vi "CoreDac.vi"(11 "Cluster":T1) -> ()   [LabVIEW 2024]
uses:
  #AquisitionLoopEnum.ctl
  <vilib>/DAQmx/create/channels.llb/DAQmx Create Channel (AI-Voltage-Basic).vi
  <vilib>/DAQmx/configure/timing.llb/DAQmx Timing (Sample Clock).vi
  <vilib>/DAQmx/read.llb/DAQmx Read (Analog 1D Wfm NChan NSamp).vi
  GUI/#GuiEnum.ctl
  GUI/#GuiQueueElement.ctl
  vision/#QueueEnum.ctl
  Correlation/#CorrelationQueueElement.ctl
  <vilib>/vision/Image Controls.llb/IMAQ Image.ctl
  Core/#CoreQueues.ctl
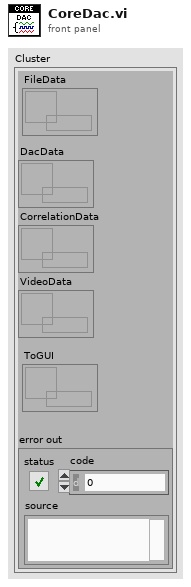
[diagram p1: front panel]
types:
  T1 = typedef "#CoreQueues.ctl" = cluster{"DacData":refnum<queue>, "CorrelationData":refnum<queue>, "VideoData":refnum<queue>, "error out":errorcluster, "ToGUI":refnum<queue>, "FileData":refnum<queue>}
  T2 = typedef "#AquisitionLoopEnum.ctl" = enum16{"Idle", "Init", "Aquisition", "End"}
  T3 = typedef "#QueueEnum.ctl" = enum16{"Ant", "Video"}
  T4 = typedef "#CorrelationQueueElement.ctl" = cluster{"Enum":T3, "t0":timestamp, dbl[]}
  T5 = typedef "#GuiEnum.ctl" = enum16{"AudioData", "VisionDistances", "DacDistances", "CorrelationDistances", "Video", "FPS"}
  T6 = typedef "#GuiQueueElement.ctl" = cluster{"Enum":T5, "Variant":variant}
  T7 = typedef "#AquisitionParameter.ctl" = cluster{"SampleRate":dbl, "BufferSize":i32, "Channels":tag}
  T8 = typedef "Sound Data Format.ctl" = cluster{"sample rate (S/s)":dbl, "number of channels":i32, "bits per sample":i32}
  T9 = cluster{"AquisitionParameters":T7, "SoundFormat":T8, "Signal type":enum16{"Sine Wave", "Triangle Wave", "Square Wave", "Sawtooth Wave"}, "Amplitude":dbl, "AudioBuffer":i32, "ChannelBounds":cluster{"InputMin":dbl, "InputMax":dbl, "OutputMin":dbl, "OutputMax":dbl}[], "MasterOffset":dbl}
  T10 = cluster{"InputMin":dbl, "InputMax":dbl, "OutputMin":dbl, "OutputMax":dbl}[]
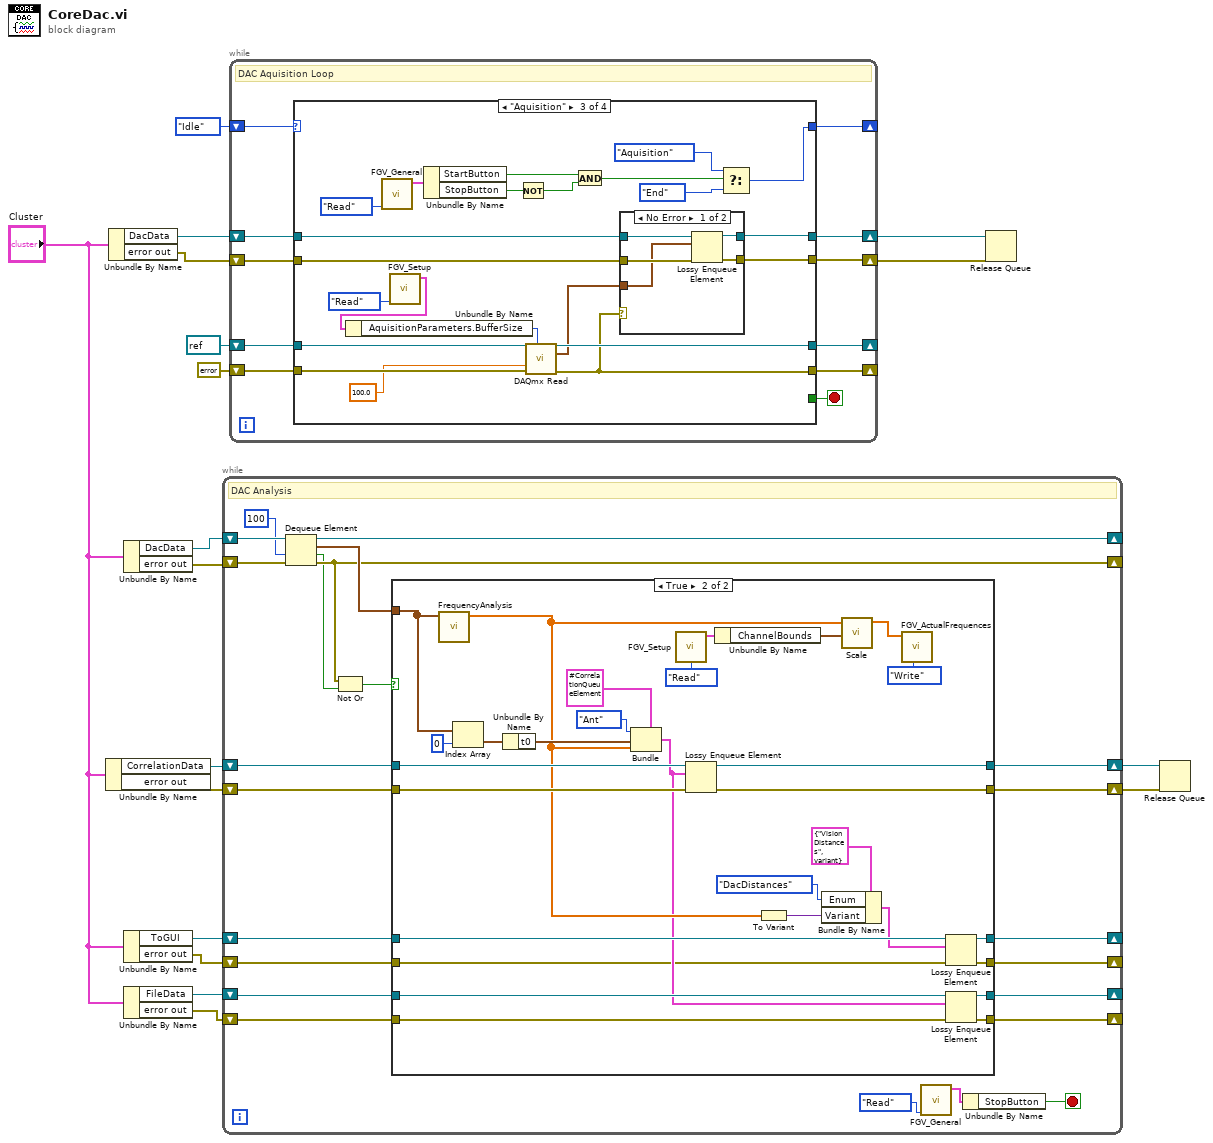
[diagram p0: block diagram]
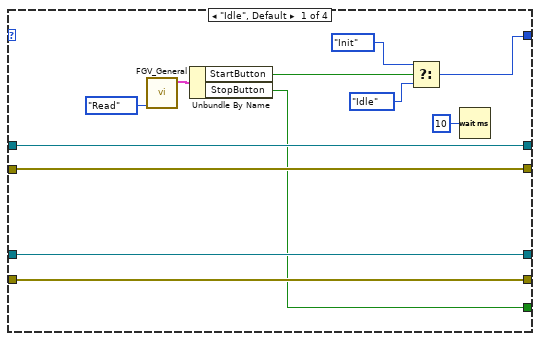
[diagram p3: hidden frame]
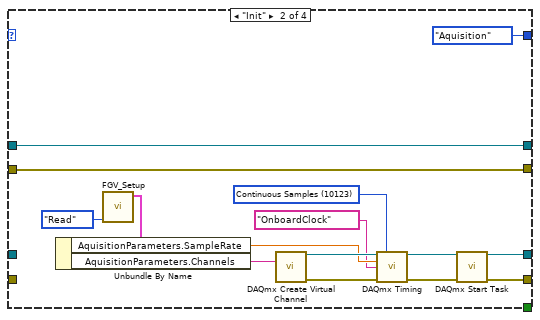
[diagram p4: hidden frame]
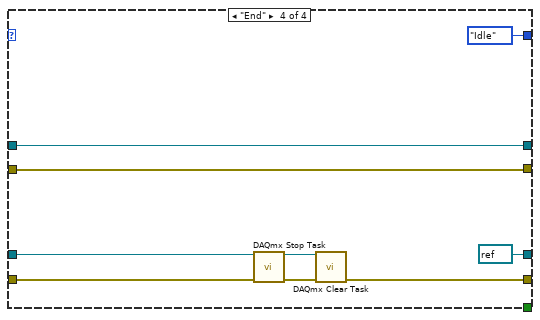
[diagram p6: hidden frame]
diagram:
  n1 = Unbundle By Name("Cluster") -> ("CorrelationData"=w9:refnum<queue>, "error out"=w8:errorcluster)
  n2 = Unbundle By Name("Cluster") -> ("DacData"=w12:refnum<queue>, "error out"=w13:errorcluster)
  n3 = Unbundle By Name("Cluster") -> ("DacData"=w7:refnum<queue>, "error out"=w6:errorcluster)
  n4 = Unbundle By Name("Cluster") -> ("ToGUI"=w10:refnum<queue>, "error out"=w11:errorcluster)
  n5 = Unbundle By Name("Cluster") -> ("FileData"=w2:refnum<queue>, "error out"=w1:errorcluster)
  n6 = while {
    shift-right: [w35] -> _
    shift-left: w6 -> [w40]
    shift-right: [w39] -> _
    shift-left: w7 -> [w41]
    shift-right: [w31] -> w4
    shift-left: w9 -> [w33]
    shift-right: [w30] -> w5
    shift-left: w8 -> [w32]
    shift-right: [w25] -> _
    shift-left: w10 -> [w26]
    shift-right: [w23] -> _
    shift-left: w11 -> [w24]
    shift-right: [w21] -> _
    shift-left: w2 -> [w22]
    shift-right: [w20] -> _
    shift-left: w1 -> [w19]
    stop <- w27 stop-if-true
    # "DAC Analysis"
    n7 = Dequeue Element(queue=w41, timeout in ms (-1)=100, error in (no error)=w40) -> (queue out=w39:refnum<queue>, element=w37:waveform(dbl)[], timed out?=w34:bool, error out=w35:errorcluster)
    n8 = Not Or(1:w34, 2:w35) -> (0:w36:bool)
    n9 = case shown="True" w36 {
      tunnel: w37 -> [_ w72]
      tunnel: w33 -> [w47 w76]
      tunnel: w32 -> [w46 w75]
      tunnel: [w47 w74] -> w31
      tunnel: [w46 w73] -> w30
      tunnel: [w44 w64] -> w25
      tunnel: w26 -> [w44 w63]
      tunnel: w24 -> [w45 w48]
      tunnel: [w45 w62] -> w23
      tunnel: w22 -> [w43 w55]
      tunnel: [w43 w54] -> w21
      tunnel: [w42 w53] -> w20
      tunnel: w19 -> [w42 w52]
      frame False {
      }
      frame True {
        n10 = call "FrequencyAnalysis.vi"("Input"=w72) -> ("Frequencies"=w56:dbl[])  [unwired: 10 in]
        n11 = Index Array(array=w72, index=0) -> (element=w70:waveform(dbl))
        n12 = Unbundle By Name(w70) -> ("t0"=w69:timestamp)
        n13 = Bundle(cluster=T4 {"Enum"=enum."Video", "t0"=timestamp(0 s since 1904-01-01), []}, "Enum"=#QueueEnum."Ant", "t0"=w69, w56) -> (w49:T4)
        n14 = call "FGV_Setup.vi"("Type"=enum16{"Read", "Write"}."Read") -> ("OutSetup"=w66:T9)  [unwired: 10 in]
        n15 = Lossy Enqueue Element(queue=w76, element=w49, error in (no error)=w75) -> (queue out=w74:refnum<queue>, error out=w73:errorcluster)  [unwired: 2 out]
        n16 = Unbundle By Name(w66) -> ("ChannelBounds"=w67:T10)
        n17 = To Variant(anything=w56) -> (Variant=w58:variant)
        n18 = Bundle By Name(cluster=T6 {"Enum"=enum."VisionDistances", "Variant"=variant} ("element"), "Enum"=#GuiEnum."DacDistances", "Variant"=w58) -> (w59:T6)
        n19 = call "Scale.vi"("Params"=w67, "Frequences"=w56) -> ("ScaleFrequences"=w65:dbl[])  [unwired: 9 in]
        n20 = call "FGV_ActualFrequences.vi"("Type"=enum16{"Read", "Write"}."Write", "Frequences"=w65) -> ()  [unwired: 9 in, 1 out]
        n21 = Lossy Enqueue Element(queue=w63, element=w59, error in (no error)=w48) -> (queue out=w64:refnum<queue>, error out=w62:errorcluster)  [unwired: 2 out]
        n22 = Lossy Enqueue Element(queue=w55, element=w49, error in (no error)=w52) -> (queue out=w54:refnum<queue>, error out=w53:errorcluster)  [unwired: 2 out]
      }
    }
    n23 = call "FGV_General.vi"("Type"=enum16{"Read", "Write"}."Read") -> ("GeneralIndicator"=w28:cluster{"StartButton":bool, "StopButton":bool})  [unwired: 10 in]
    n24 = Unbundle By Name(w28) -> ("StopButton"=w27:bool)
  }
  n25 = while {
    shift-right: [w85] -> _
    shift-left: errorcluster {"status"=FALSE, "code"=0, "source"=""} ("error out") -> [w83]
    shift-right: [w86] -> _
    shift-left: refnum<k21> refnum ("task out") -> [w84]
    shift-right: [w77] -> _
    shift-left: #AquisitionLoopEnum."Idle" -> [w87]
    shift-right: [w80] -> w18
    shift-left: w12 -> [w81]
    shift-right: [w78] -> w17
    shift-left: w13 -> [w79]
    stop <- w82 stop-if-true
    # "DAC Aquisition Loop"
    n26 = case shown="\"Aquisition\"" w87 {
      tunnel: [w96 w111 w134 refnum<k21> refnum ("task out")] -> w86
      tunnel: [w97 w110 w121 w152] -> w85
      tunnel: w84 -> [w96 _ w136 w149]
      tunnel: w83 -> [w97 _ w135 w151]
      tunnel: [w89 _ _ _] -> w82
      tunnel: w81 -> [w94 w103 w128 w146]
      tunnel: [w94 w103 w127 w146] -> w80
      tunnel: w79 -> [w93 w104 w122 w145]
      tunnel: [w93 w104 w126 w145] -> w78
      tunnel: [w92 #AquisitionLoopEnum."Aquisition" w124 #AquisitionLoopEnum."Idle"] -> w77
      frame "Idle", Default {
        n27 = call "FGV_General.vi"("Type"=enum16{"Read", "Write"}."Read") -> ("GeneralIndicator"=w90:cluster{"StartButton":bool, "StopButton":bool})  [unwired: 10 in]
        n28 = Unbundle By Name(w90) -> ("StartButton"=w88:bool, "StopButton"=w89:bool)
        n29 = Select(t=#AquisitionLoopEnum."Init", s=w88, f=#AquisitionLoopEnum."Idle") -> (s? t:f=w92:T2)
        n30 = Wait (ms)(milliseconds to wait=u32 10) -> ()  [unwired: 1 out]
      }
      frame "Init" {
        w114 = 10123 items=["Finite Samples"=10178, "Continuous Samples"=10123, "Hardware Timed Single Point"=12522] ("sample mode")
        n31 = call "FGV_Setup.vi"("Type"=enum16{"Read", "Write"}."Read") -> ("OutSetup"=w101:T9)  [unwired: 10 in]
        n32 = Unbundle By Name(w101) -> ("AquisitionParameters.SampleRate"=w108:dbl, "AquisitionParameters.Channels"=w107:tag)
        n33 = call-poly <vilib>:"DAQmx Create Virtual Channel.vi"("physical channels"=w107) -> ("task out"=w113:refnum<k21>, "error out"=w112:errorcluster)  [unwired: 13 in]
        n34 = call-poly <vilib>:"DAQmx Timing.vi"("task/channels in"=w113, "sample mode"=w114, "rate"=w108, "source"=tag "OnboardClock", "error in"=w112) -> ("task out"=w106:refnum<k21>, "error out"=w109:errorcluster)  [unwired: 9 in]
        n35 = call <vilib>:"DAQmx Start Task.vi"("task/channels in"=w106, "error in"=w109) -> ("task out"=w111:refnum<k21>, "error out"=w110:errorcluster)  [unwired: 12 in]
      }
      frame "Aquisition" {
        n36 = call "FGV_General.vi"("Type"=enum16{"Read", "Write"}."Read") -> ("GeneralIndicator"=w119:cluster{"StartButton":bool, "StopButton":bool})  [unwired: 10 in]
        n37 = call "FGV_Setup.vi"("Type"=enum16{"Read", "Write"}."Read") -> ("OutSetup"=w115:T9)  [unwired: 10 in]
        n38 = Unbundle By Name(w115) -> ("AquisitionParameters.BufferSize"=w129:i32)
        n39 = Unbundle By Name(w119) -> ("StartButton"=w117:bool, "StopButton"=w118:bool)
        n40 = Not(x=w118) -> (.not. x?=w131:bool)
        n41 = call-poly <vilib>:"DAQmx Read.vi"("task/channels in"=w136, "number of samples per channel"=w129, "timeout"=100.0, "error in"=w135) -> ("task out"=w134:refnum<k21>, "data"=w125:waveform(dbl)[], "error out"=w121:errorcluster)  [unwired: 9 in]
        n42 = And(x=w117, y=w131) -> (x .and. y?=w130:bool)
        n43 = case shown="No Error" w121 {
          tunnel: w128 -> [w141 w142]
          tunnel: [w140 w142] -> w127
          tunnel: w122 -> [w139 w143]
          tunnel: [w138 w143] -> w126
          tunnel: w125 -> [w137 _]
          frame No Error {
            n44 = Lossy Enqueue Element(queue=w141, element=w137, error in (no error)=w139) -> (queue out=w140:refnum<queue>, error out=w138:errorcluster)  [unwired: 2 out]
          }
          frame Error {
          }
        }
        n45 = Select(t=#AquisitionLoopEnum."Aquisition", s=w130, f=#AquisitionLoopEnum."End") -> (s? t:f=w124:T2)
      }
      frame "End" {
        n46 = call <vilib>:"DAQmx Stop Task.vi"("task/channels in"=w149, "error in"=w151) -> ("task out"=w148:refnum<k21>, "error out"=w150:errorcluster)  [unwired: 12 in]
        n47 = call <vilib>:"DAQmx Clear Task.vi"("task in"=w148, "error in"=w150) -> ("error out"=w152:errorcluster)  [unwired: 13 in]
      }
    }
  }
  n48 = Release Queue(queue=w18, error in (no error)=w17) -> ()  [unwired: 1 in, 3 out]
  n49 = Release Queue(queue=w4, error in (no error)=w5) -> ()  [unwired: 1 in, 3 out]
